vi "leebinario_bloque.vi"() -> ()   [LabVIEW 2015]
panel:
  in  "Nº acel":i32
  out "T, v, UT":sgl[](array[numeric])
  out "Waveform Graph":waveform(sgl)[](graph)
  in  "Folder Path":path
  out "error out":errorcluster
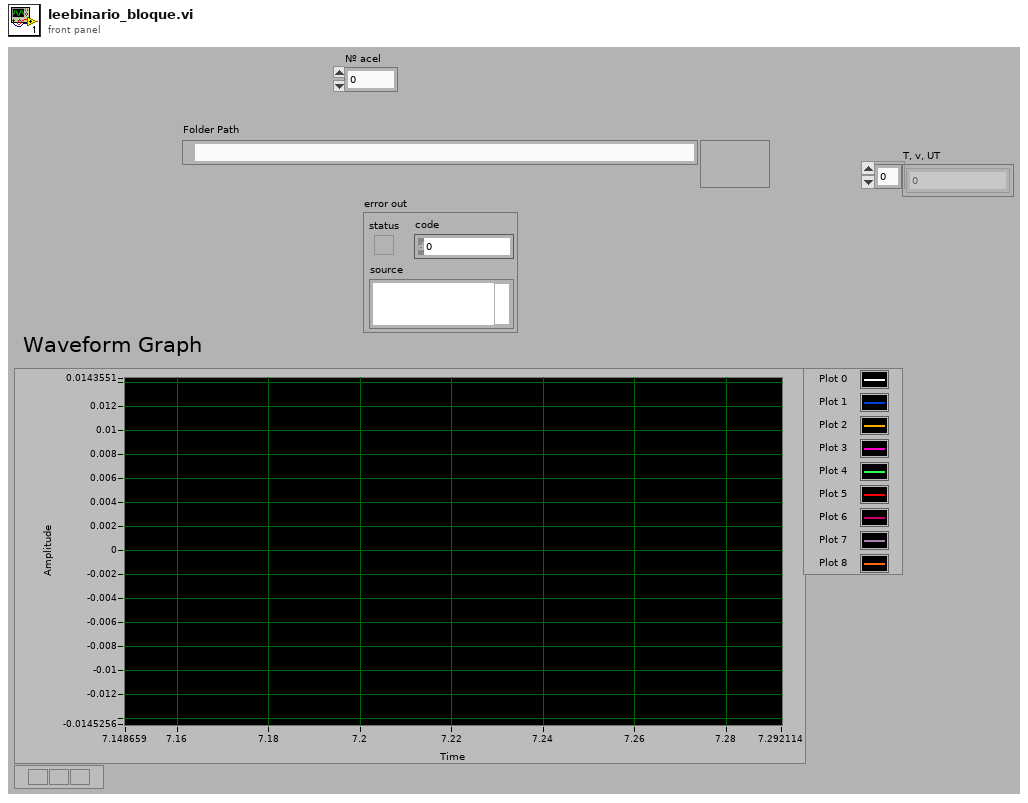
[diagram p1: front panel]
types:
  T1 = enum16{"big-endian, network order", "native, host order", "little-endian"}
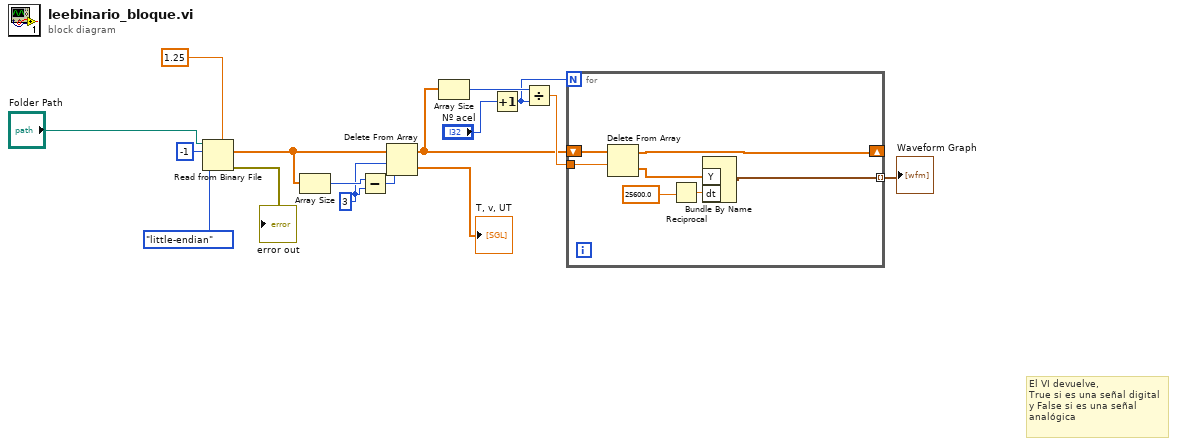
[diagram p0: block diagram]
diagram:
  w9 = 3 ("length")
  # "El VI devuelve,\nTrue si es una señal digital\ny False si es una señal\nanalógica"
  n1 = Read from Binary File(5:sgl 1.25, 9:T1."little-endian" ("byte order (0:big-endian, network order)"), 10:-1 ("count (1)"), 11:"Folder Path") -> (0:→"error out":errorcluster, 2:w8:sgl[])  [unwired: 1 in, 3 out]
  n2 = Array Size(array=w8) -> (size(s)=w11:i32)
  n3 = Subtract(x=w11, y=w9) -> (x-y=w10:i32)
  n4 = Delete From Array(array=w8, length=w9, index=w10) -> (deleted portion=→"T, v, UT":sgl[], array with subset deleted=w3:sgl[])
  n5 = Array Size(array=w3) -> (size(s)=w7:i32)
  n6 = Increment(x="Nº acel") -> (x+1=w5:i32)
  n7 = Divide(x=w7, y=w5) -> (x/y=w4:dbl)
  n8 = for {
    N: w5 -> [_]
    tunnel: [w23] -> w16 mode=indexing
    shift-right: [w19] -> _
    shift-left: w3 -> [w20]
    tunnel: w4 -> [w18]
    n9 = Delete From Array(array=w20, length=w18) -> (deleted portion=w17:sgl[], array with subset deleted=w19:sgl[])  [unwired: 1 in]
    n10 = Reciprocal(x=25600.0 ("dt")) -> (1/x=w21:dbl)
    n11 = Bundle By Name("Y"=w17, "dt"=w21) -> (w23:waveform(sgl))  [unwired: 1 in]
  }
  "Waveform Graph" <- w16
